vi "Insert Fitted Offset in Parameters Array.vi"(6 "Fitted Offset":bool, 7 "Fit Control Data in":variant, 8 "error in (no error)":errorcluster, 9 "Fixed Parameter Names in":T8[](array[typedef]), 10 "Fixed Parameter Values in":dbl[](array[numeric]), 11 "NL Fit Output in":T1={"best nonlinear fit"=[], "best fit parameters"=[], "R^2"=0.0, "RMSE"=0.0, "error out"={"status"=FALSE, "code"=0, "source"=""}, "Fitting Method"=enum."Least Square", "number of function calls"=0, "number of iterations"=0, "covariance"=[], "Chi 2"=0.0, "DOF"=0, "Fit Convergence Criterion"=enum."Continue", "Fitting Algorithm"=enum."Levenberg-Marquardt", "Weighted Fit"=enum."Unweighted", "Gradient"=0.0, "|Delta Chi 2|"=0.0, "|Delta Chi 2|/Chi 2"=0.0, "Max |Delta a| /|a|"=0.0, "Lambda"=-1.0, "RSS"=0.0, "AIC"=0.0, "BIC"=0.0, "Max number of function calls"=0, "Max number of iterations"=0, "IRF"={"X Array"=[], "Y Array"=[]}, "IRF Normalization Factor"=0.0, "Decay Normalization Factor"=0.0, "Number of offset fits"=0, "Weighted Chi2"=-1.0, "Unweighted Chi2"=-1.0}) -> (0 "error out":errorcluster, 1 "Fixed Parameter Names out":T8[](array[typedef]), 2 "Fixed Parameter Values out":dbl[](array[numeric]), 3 "NL Fit Output out":T1={"best nonlinear fit"=[], "best fit parameters"=[], "R^2"=0.0, "RMSE"=0.0, "error out"={"status"=FALSE, "code"=0, "source"=""}, "Fitting Method"=enum."Least Square", "number of function calls"=0, "number of iterations"=0, "covariance"=[], "Chi 2"=0.0, "DOF"=0, "Fit Convergence Criterion"=enum."Continue", "Fitting Algorithm"=enum."Levenberg-Marquardt", "Weighted Fit"=enum."Unweighted", "Gradient"=0.0, "|Delta Chi 2|"=0.0, "|Delta Chi 2|/Chi 2"=0.0, "Max |Delta a| /|a|"=0.0, "Lambda"=-1.0, "RSS"=0.0, "AIC"=0.0, "BIC"=0.0, "Max number of function calls"=0, "Max number of iterations"=0, "IRF"={"X Array"=[], "Y Array"=[]}, "IRF Normalization Factor"=0.0, "Decay Normalization Factor"=0.0, "Number of offset fits"=0, "Weighted Chi2"=-1.0, "Unweighted Chi2"=-1.0}, 5 "Fit Control Data out":variant)   [LabVIEW 2021, in "Fits.lvlib"]
uses:
  Fits.lvlib
  IRF(X)PSED/Decay Fit Parameters In List.ctl
  Non-linear Fit Output v4.ctl
  Nonlinear Fit Method.ctl
  <vilib>/Analysis/Matrix/Datatypes/RealMatrix.ctl
  Convergence Criteria.ctl
  Non-linear Fitting Algorithm.ctl
  IRF(X)PSED/Fit Weights Type v2.ctl
  Graphs/XY Graph/XY Graph Plot Data.ctl
  Decay Convolution/Fit Control Data v2.ctl
  Decay Convolution/Decay Model.ctl
  Graphs/XY Graph/XY Graph Add-Ons.lvlib
  <vilib>/Analysis/Matrix/NI_Matrix.lvlib
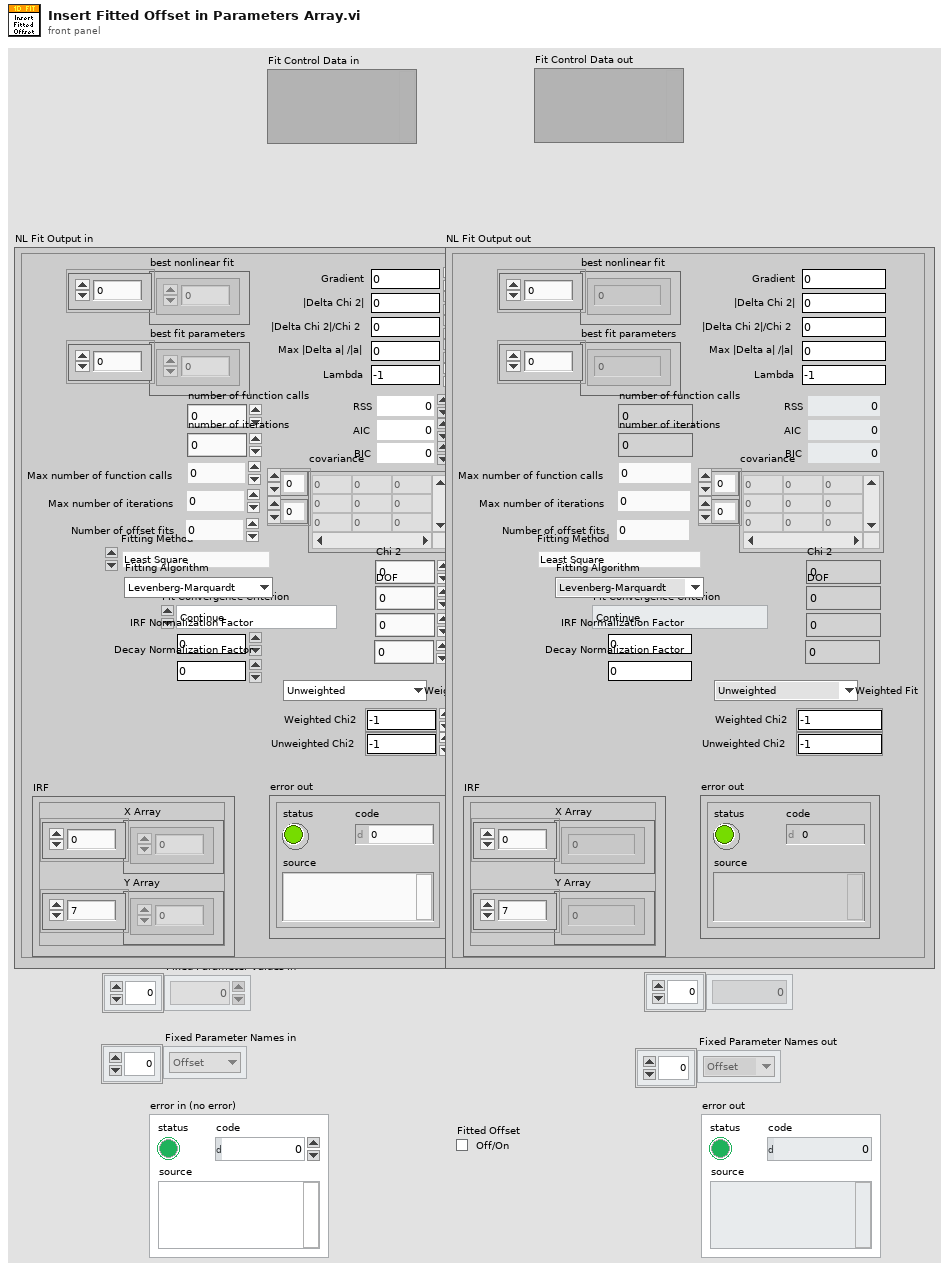
[diagram p1: front panel]
types:
  T1 = typedef "Fits.lvlib/Non-linear Fit Output v4.ctl" = cluster{"best nonlinear fit":dbl[], "best fit parameters":dbl[], "R^2":dbl, "RMSE":dbl, "error out":errorcluster, "Fitting Method":T2, "number of function calls":i32, "number of iterations":i32, "covariance":T3, "Chi 2":dbl, "DOF":i32, "Fit Convergence Criterion":T4, "Fitting Algorithm":T5, "Weighted Fit":T6, "Gradient":dbl, "|Delta Chi 2|":dbl, "|Delta Chi 2|/Chi 2":dbl, "Max |Delta a| /|a|":dbl, "Lambda":dbl, "RSS":dbl, "AIC":dbl, "BIC":dbl, "Max number of function calls":i32, "Max number of iterations":i32, "IRF":T7, "IRF Normalization Factor":dbl, "Decay Normalization Factor":dbl, "Number of offset fits":i32, "Weighted Chi2":dbl, "Unweighted Chi2":dbl}
  T2 = typedef "Fits.lvlib/Nonlinear Fit Method.ctl" = enum16{"Least Square", "Least Absolute Residual", "Bisquare", "MLE"}
  T3 = typedef "NI_Matrix.lvlib/RealMatrix.ctl" = dbl[][]
  T4 = typedef "Fits.lvlib/Convergence Criteria.ctl" = enum16{"Continue", "Tolerances Exceeded", "Max Time Exceeded", "Max Iterations Exceeded", "Max Function Evaluations Exceeded", "Scale Range Exceeded"}
  T5 = typedef "Fits.lvlib/Non-linear Fitting Algorithm.ctl" = enum16{"Levenberg-Marquardt", "Trust-Region Dogleg"}
  T6 = typedef "Fits.lvlib/Fit Weights Type v2.ctl" = enum16{"Unweighted", "1/Variance (Neyman)", "1/Variance (Pearson)", "Best of All"}
  T7 = typedef "XY Graph Add-Ons.lvlib/XY Graph Plot Data.ctl" = cluster{"X Array":dbl[], "Y Array":dbl[]}
  T8 = typedef "Fits.lvlib/Decay Fit Parameters In List.ctl" = enum16{"Offset", "Baseline", "A_1", "tau_1", "A_2", "tau_2"}
  T9 = typedef "Fits.lvlib/Fit Control Data v2.ctl" = cluster{"IRF":T7, "Laser Period":dbl, "SYNC Period":dbl, "Fixed Parameter Names":T8[], "Fixed Parameter Values":dbl[], "Fitted Parameter Names":T8[], "Fit Model":T10}
  T10 = typedef "Fits.lvlib/Decay Model.ctl" = enum16{"1-Exponential", "2-Exponentials"}
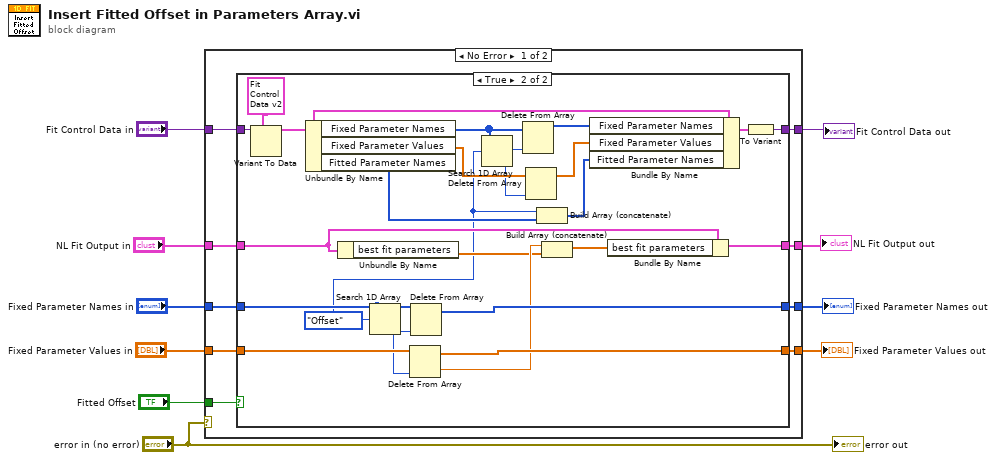
[diagram p0: block diagram]
diagram:
  n1 = case shown="No Error" "error in (no error)" {
    tunnel: "Fitted Offset" -> [w19 _]
    tunnel: "Fixed Parameter Names in" -> [w18 w50]
    tunnel: [w17 w50] -> w8
    tunnel: "Fixed Parameter Values in" -> [w16 w49]
    tunnel: [w15 w49] -> w6
    tunnel: "NL Fit Output in" -> [w14 w48]
    tunnel: [w13 w48] -> w3
    tunnel: "Fit Control Data in" -> [w12 w47]
    tunnel: [w11 w47] -> w1
    frame No Error {
      n2 = case shown="True" w19 {
        tunnel: w18 -> [w23 w44]
        tunnel: [w23 w42] -> w17
        tunnel: w16 -> [w22 w46]
        tunnel: [w22 w45] -> w15
        tunnel: w14 -> [w21 w38]
        tunnel: [w21 w40] -> w13
        tunnel: w12 -> [w20 w35]
        tunnel: [w20 w24] -> w11
        frame False {
        }
        frame True {
          w27 = Decay_Fit_Parameters_In_List."Offset" ("element")
          n3 = Variant To Data(type=T9 {"IRF"={"X Array"=[], "Y Array"=[]}, "Laser Period"=0.0, "SYNC Period"=0.0, "Fixed Parameter Names"=[], "Fixed Parameter Values"=[], "Fitted Parameter Names"=[], "Fit Model"=enum."1-Exponential"} ("Fit Control Data"), Variant=w35) -> (data=w26:T9)  [unwired: 1 in, 1 out]
          n4 = Unbundle By Name(w26) -> ("Fixed Parameter Names"=w36:T8[], "Fixed Parameter Values"=w33:dbl[], "Fitted Parameter Names"=w29:T8[])
          n5 = Unbundle By Name(w38) -> ("best fit parameters"=w37:dbl[])
          n6 = Search 1D Array(1D array=w44, element=w27) -> (index of element=w43:i32)  [unwired: 1 in]
          n7 = Delete From Array(array=w46, index=w43) -> (deleted portion=w41:dbl, array with subset deleted=w45:dbl[])  [unwired: 1 in]
          n8 = Delete From Array(array=w44, index=w43) -> (array with subset deleted=w42:T8[])  [unwired: 1 in, 1 out]
          n9 = Search 1D Array(1D array=w36, element=w27) -> (index of element=w31:i32)  [unwired: 1 in]
          n10 = Delete From Array(array=w36, index=w31) -> (array with subset deleted=w34:T8[])  [unwired: 1 in, 1 out]
          n11 = Delete From Array(array=w33, index=w31) -> (array with subset deleted=w32:dbl[])  [unwired: 1 in, 1 out]
          n12 = Build Array (concatenate)(w27, w29) -> (w28:T8[])
          n13 = Build Array (concatenate)(w41, w37) -> (w39:dbl[])
          n14 = Bundle By Name(cluster=w26, "Fixed Parameter Names"=w34, "Fixed Parameter Values"=w32, "Fitted Parameter Names"=w28) -> (w30:T9)
          n15 = Bundle By Name(cluster=w38, "best fit parameters"=w39) -> (w40:T1)
          n16 = To Variant(anything=w30) -> (Variant=w24:variant)
        }
      }
    }
    frame Error {
    }
  }
  "Fixed Parameter Names out" <- w8
  "Fixed Parameter Values out" <- w6
  "NL Fit Output out" <- w3
  "Fit Control Data out" <- w1
  "error out" <- "error in (no error)"
